vi "SP Convert De-Embed Cluster.vi"(4 "Fields Names":string[](array[string]), 5 "Conversion":enum16{"Cluster - HTML", "HTML - Cluster"}(ring), 7 "De-Embed Key Array In":T4, 8 "De-Embed Cluster In":T1={"De-Embed"=TRUE, "Adapters"=[]}) -> (1 "De-Embed Cluster Out":T1={"De-Embed"=TRUE, "Adapters"=[]}, 2 "Measurements HTML Out":string)   [LabVIEW 2011]
uses:
  ITK/utils/keyedarr.llb/Keyed Array.ctl
  TypeDefs/SP De-Embed.ctl
  TypeDefs/SP Adapter.ctl
  TypeDefs/SP Data.ctl
  ITK/utils/strutil.llb/Case Matching.ctl
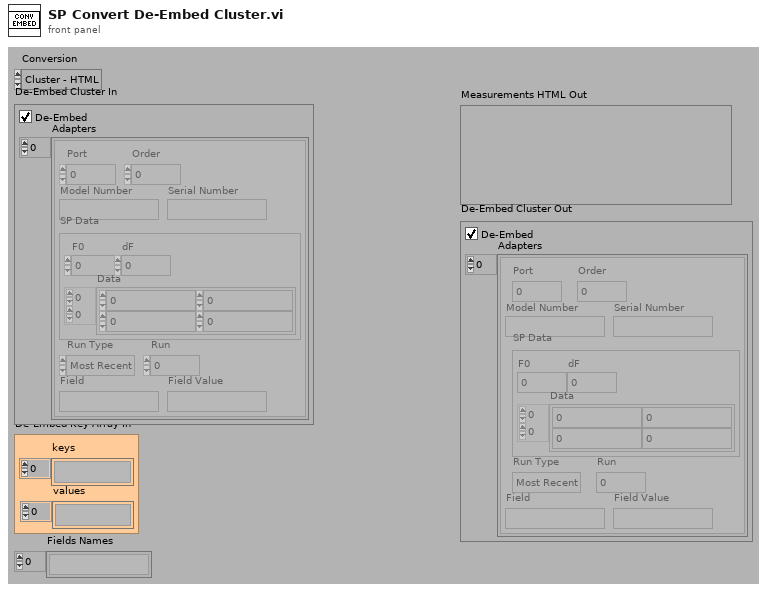
[diagram p1: front panel]
types:
  T1 = typedef "SP De-Embed.ctl" = cluster{"De-Embed":bool, "Adapters":T2[]}
  T2 = typedef "SP Adapter.ctl" = cluster{"Port":i8, "Order":i8, "Model Number":string, "Serial Number":string, "SP Data":T3, "Run Type":enum16{"Most Recent", "Run #", "Match Field"}, "Run":i32, "Field":string, "Field Value":string}
  T3 = typedef "SP Data.ctl" = cluster{"F0":dbl, "dF":dbl, "Data":cdb[][]}
  T4 = typedef "Keyed Array.ctl" = cluster{"keys":string[], "values":string[]}
  T5 = typedef "Case Matching.ctl" = enum16{"a != A", "a == A", "system"}
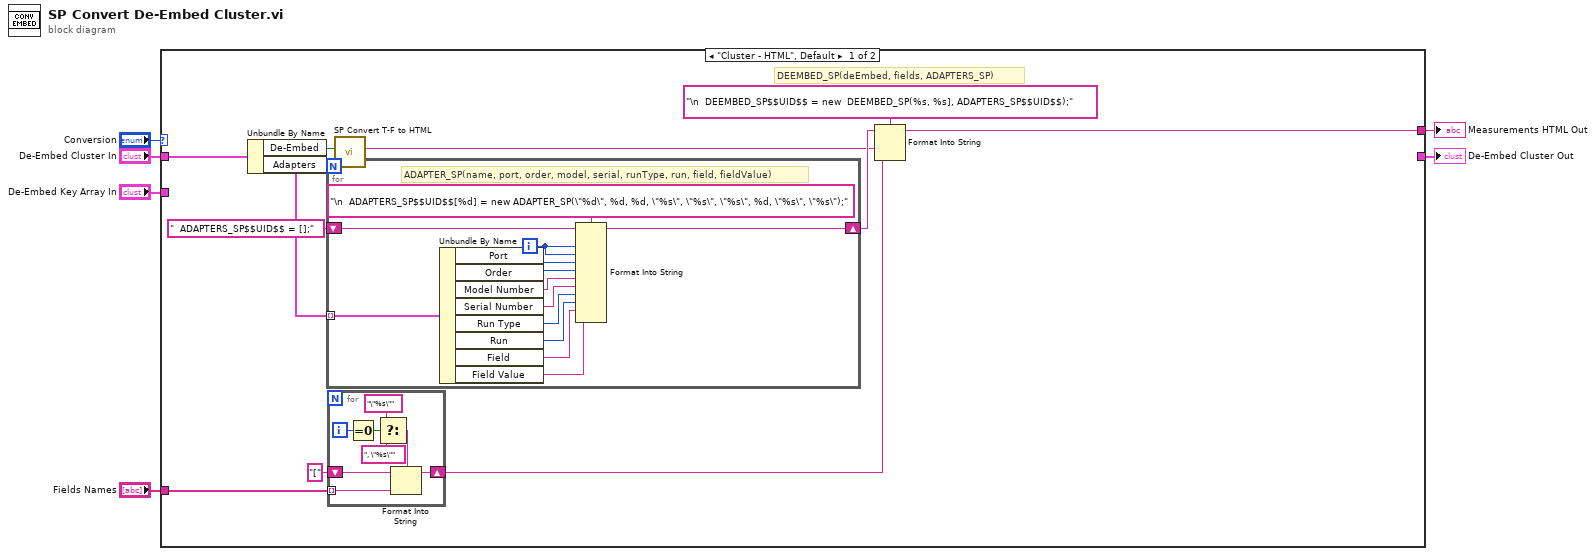
[diagram p0: block diagram]
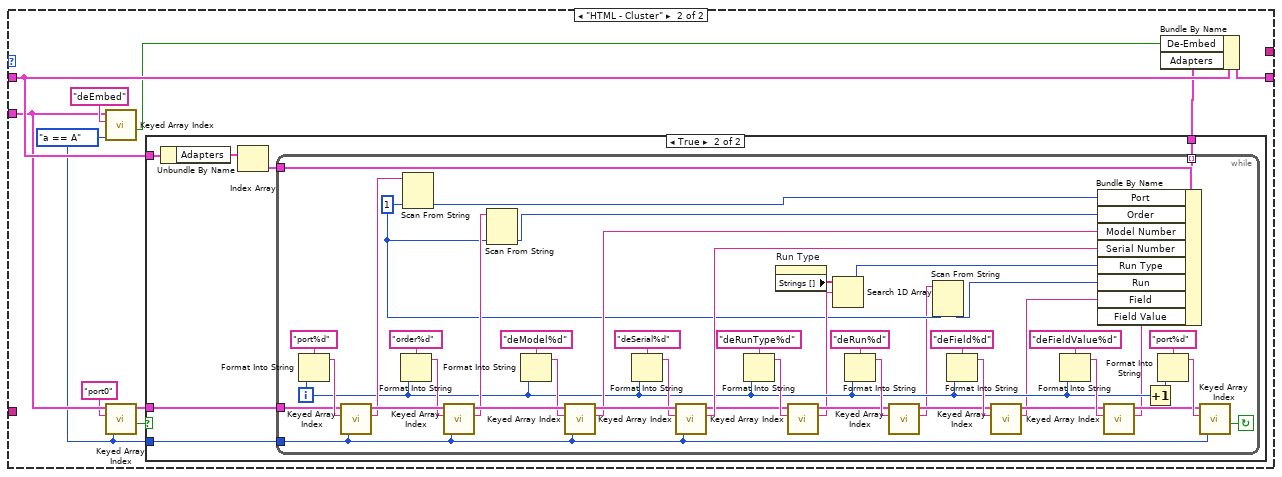
[diagram p2: hidden frame]
diagram:
  n1 = case shown="\"Cluster - HTML\", Default" "Conversion" {
    tunnel: "De-Embed Cluster In" -> [w17 w47]
    tunnel: "De-Embed Key Array In" -> [_ w43]
    tunnel: [w12 _] -> w3
    tunnel: [_ w45] -> w2
    tunnel: "Fields Names" -> [w7 _]
    frame "Cluster - HTML", Default {
      # "DEEMBED_SP(deEmbed, fields, ADAPTERS_SP)"
      n2 = Unbundle By Name(w17) -> ("De-Embed"=w15:bool, "Adapters"=w13:T2[])
      n3 = for {
        tunnel: w13 -> [w38] mode=indexing
        shift-right: [w33] -> w11
        shift-left: "  ADAPTERS_SP$$UID$$ = [];" ("format string") -> [w32]
        i -> [w31]
        # "ADAPTER_SP(name, port, order, model, serial, runType, run, field, fieldValue)"
        n4 = Unbundle By Name(w38) -> ("Port"=w35:i8, "Order"=w34:i8, "Model Number"=w36:string, "Serial Number"=w30:string, "Run Type"=w28:enum16{"Most Recent", "Run #", "Match Field"}, "Run"=w27:i32, "Field"=w26:string, "Field Value"=w29:string)
        n5 = Format Into String(format string="\n  ADAPTERS_SP$$UID$$[%d] = new ADAPTER_SP(\"%d\", %d, %d, \"%s\", \"%s\", \"%s\", %d, \"%s\", \"%s\");", initial string=w32, w31, w31, w35, w34, w36, w30, w28, w27, w26, w29) -> (resulting string=w33:string)  [unwired: 1 in, 1 out]
      }
      n6 = for {
        shift-right: [w18] -> w8
        shift-left: "[" ("format string") -> [w25]
        tunnel: w7 -> [w19] mode=indexing
        i -> [w24]
        n7 = Equal To 0?(x=w24) -> (x = 0?=w23:bool)
        n8 = Select(t="\"%s\"" ("format string"), s=w23, f=", \"%s\"" ("format string")) -> (s? t:f=w20:string)
        n9 = Format Into String(format string=w20, initial string=w25, w19) -> (resulting string=w18:string)  [unwired: 1 in, 1 out]
      }
      n10 = call "SP Convert T-F to HTML.vi"("(T/F)"=w15) -> ("HTML (true/false)"=w10:string)  [unwired: 10 out]
      n11 = Format Into String(format string="\n  DEEMBED_SP$$UID$$ = new  DEEMBED_SP(%s, %s], ADAPTERS_SP$$UID$$);", initial string=w11, w10, w8) -> (resulting string=w12:string)  [unwired: 1 in, 1 out]
    }
    frame "HTML - Cluster" {
      w41 = Case_Matching."a == A" ("case matching (sensitive)")
      n12 = call "Keyed Array Index.vi"("case matching (sensitive)"=w41, "key"="deEmbed", "array in"=w43) -> ("valid key"=w44:bool)  [unwired: 1 in, 3 out]
      n13 = call "Keyed Array Index.vi"("case matching (sensitive)"=w41, "key"="port0", "array in"=w43) -> ("valid key"=w39:bool, "duplicate array"=w42:T4)  [unwired: 1 in, 2 out]
      n14 = case shown="True" w39 {
        tunnel: w47 -> [_ w54]
        tunnel: [_ w51] -> w46
        tunnel: w42 -> [_ w50]
        tunnel: w41 -> [_ w49]
        frame False {
        }
        frame True {
          n15 = Unbundle By Name(w54) -> ("Adapters"=w52:T2[])
          n16 = Index Array(array=w52) -> (element=w53:T2)  [unwired: 1 in]
          n17 = while {
            tunnel: w53 -> [w99]
            tunnel: w49 -> [w77]
            tunnel: [w84] -> w51 mode=indexing
            tunnel: w50 -> [w83]
            i -> [w63]
            stop <- w85 continue-if-true
            w59 = i8 1 ("default value 1")
            n18 = Format Into String(format string="port%d", w63) -> (resulting string=w97:string)  [unwired: 2 in, 1 out]
            n19 = call "Keyed Array Index.vi"("case matching (sensitive)"=w77, "key"=w97, "array in"=w83) -> ("value"=w96:string, "duplicate array"=w100:T4)  [unwired: 1 in, 2 out]
            n20 = Format Into String(format string="order%d", w63) -> (resulting string=w92:string)  [unwired: 2 in, 1 out]
            n21 = Scan From String(input string=w96, default 1=w59) -> (output 1=w95:i8)  [unwired: 3 in, 3 out]
            n22 = call "Keyed Array Index.vi"("case matching (sensitive)"=w77, "key"=w92, "array in"=w100) -> ("value"=w90:string, "duplicate array"=w101:T4)  [unwired: 1 in, 2 out]
            n23 = Scan From String(input string=w90, default 1=w59) -> (output 1=w89:i8)  [unwired: 3 in, 3 out]
            n24 = Format Into String(format string="deModel%d", w63) -> (resulting string=w91:string)  [unwired: 2 in, 1 out]
            n25 = call "Keyed Array Index.vi"("case matching (sensitive)"=w77, "key"=w91, "array in"=w101) -> ("value"=w79:string, "duplicate array"=w81:T4)  [unwired: 1 in, 2 out]
            n26 = Format Into String(format string="deSerial%d", w63) -> (resulting string=w80:string)  [unwired: 2 in, 1 out]
            n27 = call "Keyed Array Index.vi"("case matching (sensitive)"=w77, "key"=w80, "array in"=w81) -> ("value"=w78:string, "duplicate array"=w68:T4)  [unwired: 1 in, 2 out]
            n28 = Format Into String(format string="deRunType%d", w63) -> (resulting string=w76:string)  [unwired: 2 in, 1 out]
            n29 = property on="Run Type" class="Enum (strict)"() -> ("Strings []"=w62:string[])  [unwired: 2 in, 2 out]
            n30 = call "Keyed Array Index.vi"("key"=w76, "array in"=w68) -> ("value"=w61:string, "duplicate array"=w67:T4)  [unwired: 2 in, 2 out]
            n31 = Search 1D Array(1D array=w62, element=w61) -> (index of element=w60:i32)  [unwired: 1 out]
            n32 = Format Into String(format string="deRun%d", w63) -> (resulting string=w73:string)  [unwired: 2 in, 1 out]
            n33 = call "Keyed Array Index.vi"("key"=w73, "array in"=w67) -> ("value"=w58:string, "duplicate array"=w66:T4)  [unwired: 2 in, 2 out]
            n34 = Scan From String(input string=w58, default 1=w59) -> (output 1=w57:i8)  [unwired: 3 in, 3 out]
            n35 = Format Into String(format string="deField%d", w63) -> (resulting string=w72:string)  [unwired: 2 in, 1 out]
            n36 = call "Keyed Array Index.vi"("key"=w72, "array in"=w66) -> ("value"=w56:string, "duplicate array"=w65:T4)  [unwired: 2 in, 2 out]
            n37 = Format Into String(format string="deFieldValue%d", w63) -> (resulting string=w69:string)  [unwired: 2 in, 1 out]
            n38 = call "Keyed Array Index.vi"("key"=w69, "array in"=w65) -> ("value"=w55:string, "duplicate array"=w64:T4)  [unwired: 2 in, 2 out]
            n39 = Bundle By Name(cluster=w99, "Port"=w95, "Order"=w89, "Model Number"=w79, "Serial Number"=w78, "Run Type"=w60, "Run"=w57, "Field"=w56, "Field Value"=w55) -> (w84:T2)
            n40 = Increment(x=w63) -> (x+1=w87:i32)
            n41 = Format Into String(format string="port%d", w87) -> (resulting string=w86:string)  [unwired: 2 in, 1 out]
            n42 = call "Keyed Array Index.vi"("case matching (sensitive)"=w77, "key"=w86, "array in"=w64) -> ("valid key"=w85:bool)  [unwired: 1 in, 3 out]
          }
        }
      }
      n43 = Bundle By Name(cluster=w47, "De-Embed"=w44, "Adapters"=w46) -> (w45:T1)
    }
  }
  "Measurements HTML Out" <- w3
  "De-Embed Cluster Out" <- w2
